vi "OneView.vi"() -> ()   [LabVIEW 2014]
uses:
  <vilib>/Utility/inputDevices.llb/keyboardAcquire.vi
  <vilib>/picture/3D Picture Control/NI_3D Picture Control.lvlib
  <vilib>/picture/3D Picture Control/Object/Create Object (name).vi
panel:
  out "View":refnum<vi>(3d-picture)
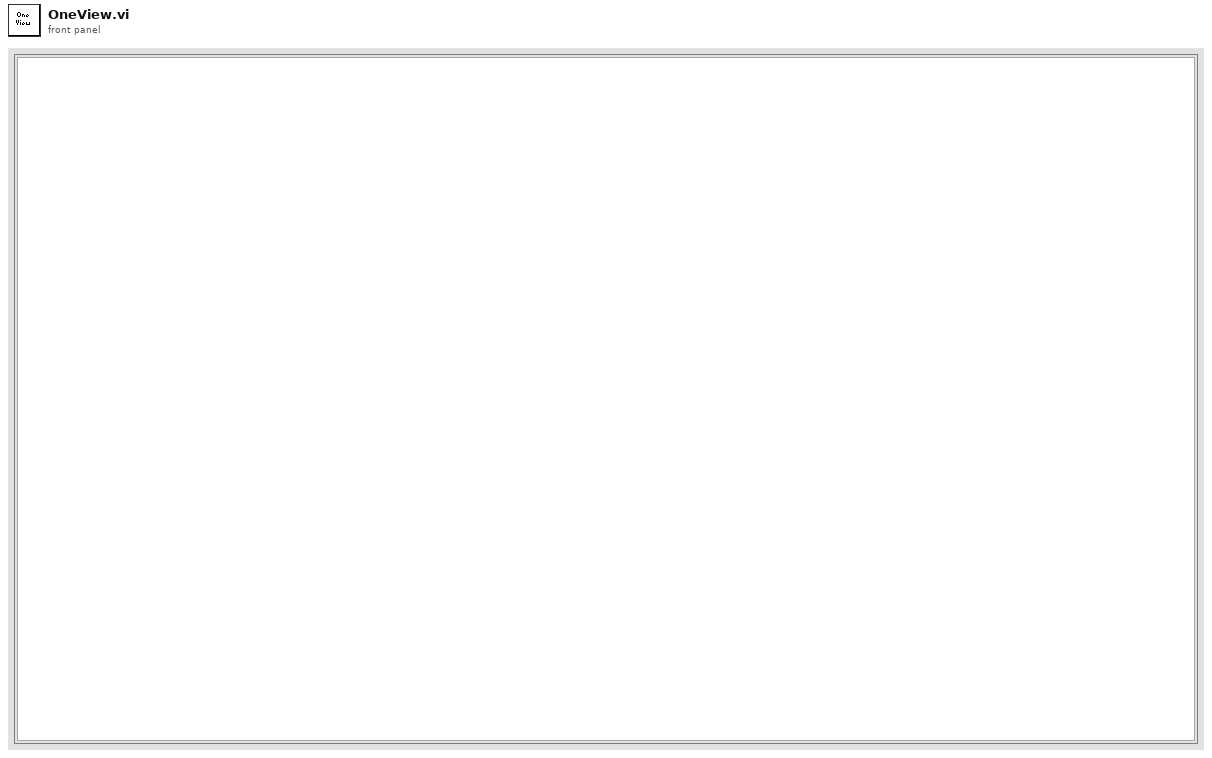
[diagram p1: front panel]
types:
  T1 = enum16{"None", "Spherical", "Flying", "Oriented"}
  T2 = enum16{"0", "1", "2", "3", "4", "5", "6", "7", "8", "9", "A", "B", "C", "D", "E", "F", "G", "H", "I", "J", "K", "L", "M", "N", "O", "P", "Q", "R", "S", "T", "U", "V", "W", "X", "Y", "Z", "F1", "F2", "F3", "F4", "F5", "F6", "F7", "F8", "F9", "F10", "F11", "F12", "F13", "F14", "F15", "ADD", "BACK", "BACKSLASH", "CAPITAL", "COMMA", "DECIMAL", "DELETE", "DIVIDE", "DOWN", "END", "EQUALS", "ESCAPE", "GRAVE (`)", "HOME", "INSERT", "LBRACKET", "LCONTROL", "LEFT", "L ALT", "LSHIFT", "LWIN", "MINUS", "MULTIPLY", "NEXT", "NUMLOCK", "NUMPAD_0", "NUMPAD_1", "NUMPAD_2", "NUMPAD_3", "NUMPAD_4", "NUMPAD_5", "NUMPAD_6", "NUMPAD_7", "NUMPAD_8", "NUMPAD_9", "PAUSE", "PERIOD", "PRIOR (PG UP)", "RBRACKET", "RCONTROL", "RETURN", "RIGHT", "R ALT", "RSHIFT", "RWIN", "SCROLL", "SEMICOLON", "SLASH", "SPACE", "SUBTRACT", "TAB", "UP", "ENTER (num pad)", "' (quote)"}
  T3 = typedef "lveventtype.ctl" = enum32{"Null", "Timeout", "Annotation Menu Selection", "Annotation Menu Selection?", "App Instance Close", "App Instance Close?", "Autoscale Range Change", "Bookmark Info Change", "Cell Edit", "Cell Edit?", "Cursor Grab", "Cursor Grab?", "Cursor Menu Selection", "Cursor Menu Selection?", "Cursor Move", "Cursor Release", "Data Change", "Direction Change", "Display State Change", "Drag Ended", "Drag Enter", "Drag Leave", "Drag Over", "Drag Source Update", "Drag Starting", "Drag Starting?", "Drop", "Exec State Change", "Key Down", "Key Down?", "Key Repeat", "Key Repeat?", "Key Up", "Listbox Double Click", "Menu Activation?", "Menu Selection (App)", "Menu Selection? (App)", "Menu Selection (User)", "Mouse Down", "Mouse Down?", "Mouse Enter", "Mouse Leave", "Mouse Move", "Mouse Up", "Mouse Wheel", "NI Security User Change (App)", "Pane Size", "Panel Close", "Panel Close?", "Panel Resize", "Plot Attribute Change", "Scale Range Change", "Shortcut Menu Activation?", "Shortcut Menu Selection (App)", "Shortcut Menu Selection? (App)", "Shortcut Menu Selection (User)", "Tree Double Click", "Tree Drag", "Tree Drag?", "Tree Drop", "Tree Drop?", "Tree Item Close", "Tree Item Close?", "Tree Item Open", "Tree Item Open?", "User Event", "Value Change"}
  T4 = typedef "LVPoint32TypeDef.ctl" = cluster{"Horizontal":i32, "Vertical":i32}
  T5 = enum16{"0", "1", "2", "3", "4", "5", "6", "7", "8", "9", "A", "B", "C", "D", "E", "F", "G", "H", "I", "J", "K", "L", "M", "N", "O", "P", "Q", "R", "S", "T", "U", "V", "W", "X", "Y", "Z", "F1", "F2", "F3", "F4", "F5", "F6", "F7", "F8", "F9", "F10", "F11", "F12", "F13", "F14", "F15", "ADD", "BACK", "BACKSLASH", "CAPITAL", "COMMA", "DECIMAL", "DELETE", "DIVIDE", "DOWN", "END", "EQUALS", "ESCAPE", "GRAVE (`)", "HOME", "INSERT", "LBRACKET", "LCONTROL", "LEFT", "L ALT", "LSHIFT", "LWIN", "MINUS", "MULTIPLY", "NEXT", "NUMLOCK", "NUMPAD_0", "NUMPAD_1", "NUMPAD_2", "NUMPAD_3", "NUMPAD_4", "NUMPAD_5", "NUMPAD_6", "NUMPAD_7", "NUMPAD_8", "NUMPAD_9", "PAUSE", "PERIOD", "PRIOR (PG UP)", "RBRACKET", "RCONTROL", "RETURN", "RIGHT", "R ALT", "RSHIFT", "RWIN", "SCROLL", "SEMICOLON", "SLASH", "SPACE", "SUBTRACT", "TAB", "UP", "ENTER (num pad)", "' (quote)"}[]
  T6 = typedef "Camera.ctl" = cluster{"Camera Position":T7, "Target":T7, "Up Direction":T7}
  T7 = typedef "LV3DPointTypeDef.ctl" = cluster{"X":sgl, "Y":sgl, "Z":sgl}
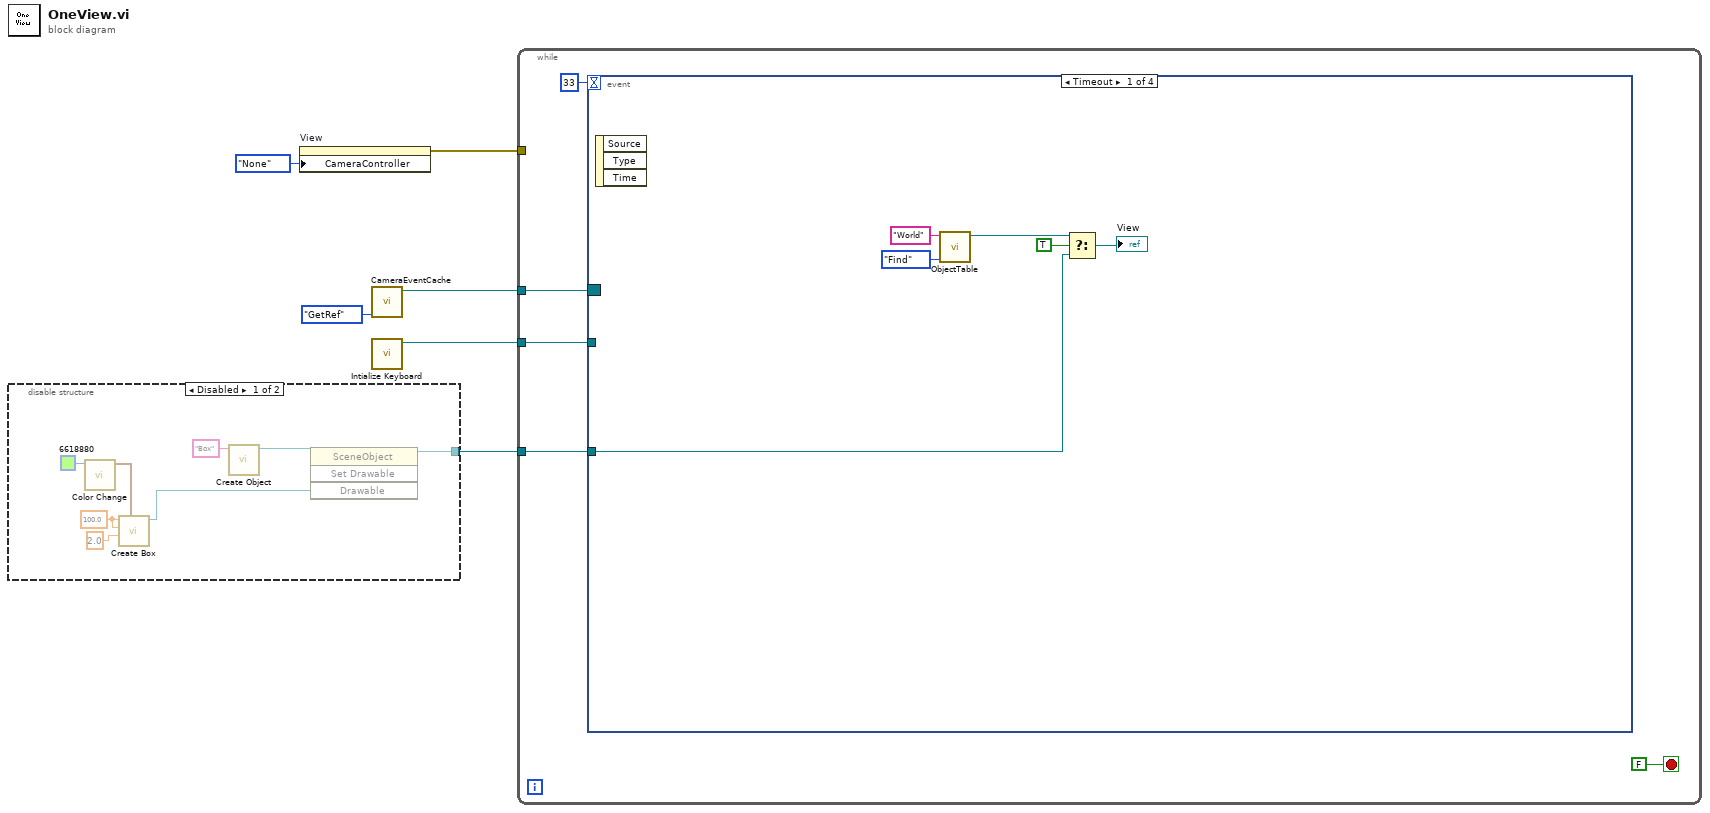
[diagram p0: block diagram]
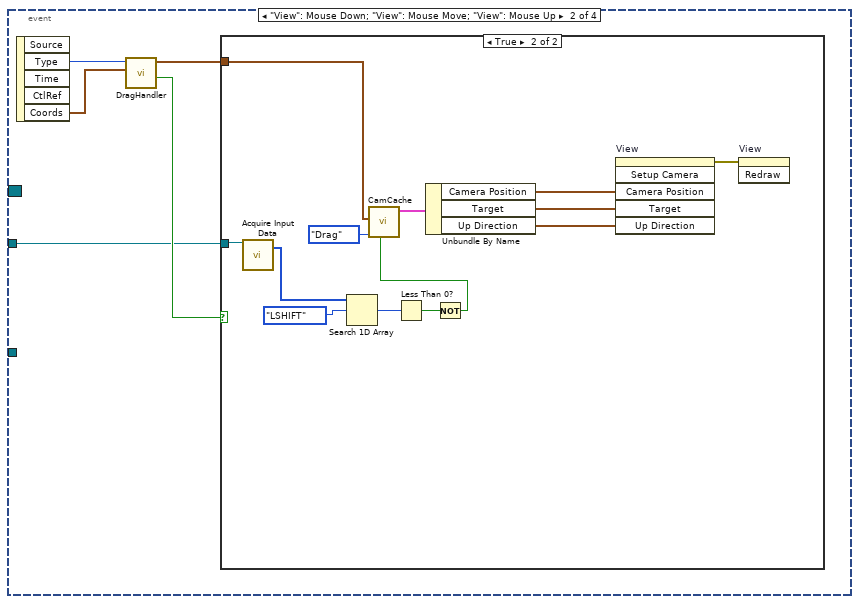
[diagram p3: hidden frame]
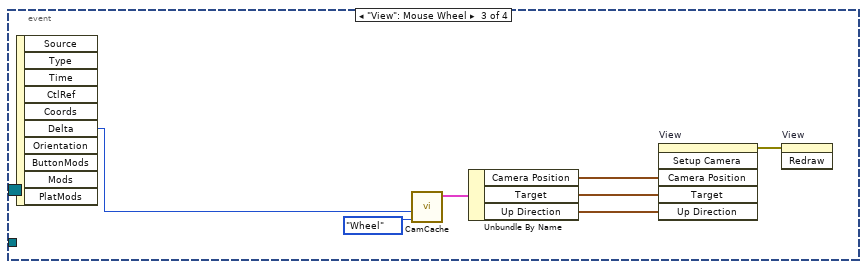
[diagram p5: hidden frame]
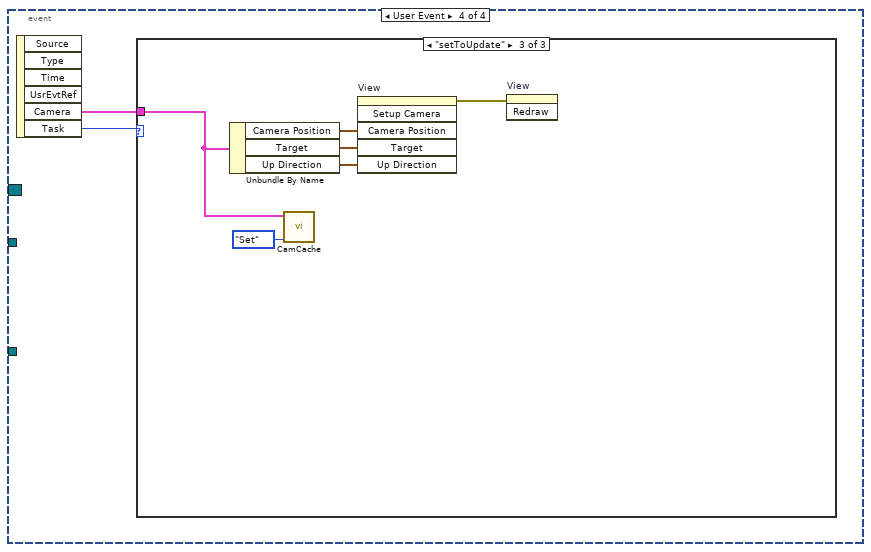
[diagram p6: hidden frame]
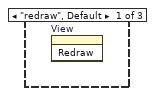
[diagram p7: hidden frame]
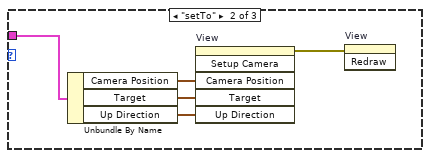
[diagram p8: hidden frame]
diagram:
  n1 = disable-structure shown="Disabled" {
    disable-tunnel: [w7 _] -> w4
    frame Disabled {
      w14 = sgl 100.0 ("Length X")
      n2 = call <vilib>:"Color Change.vi"("Color"=u32 6618880) -> ("RGBA"=w11:cluster{"R":sgl, "G":sgl, "B":sgl, "A":sgl})  [unwired: 10 in]
      n3 = call <vilib>:"Create Box.vi"("Color"=w11, "Length Z"=sgl 2.0, "Length Y"=w14, "Length X"=w14) -> ("New Box Refnum"=w8:refnum<vi>)  [unwired: 6 in, 1 out]
      n4 = call-poly <vilib>:"Create Object.vi"("Name"="Box") -> ("Scene:New Object"=w9:refnum<vi>)  [unwired: 9 in, 1 out]
      n5 = invoke class="SceneObject" method="Set Drawable"(reference=w9, "Drawable"=w8) -> (reference out=w7:refnum<vi>)  [unwired: 2 in, 3 out]
    }
    frame Enabled {
    }
  }
  n6 = property on="View" class="SceneGraphDisp (strict)"("CameraController"=T1."None" ("Camera Controller:Type")) -> (error out=w5:errorcluster)  [unwired: 2 in, 1 out]
  n7 = call "CameraEventCache.vi"("Operation"=enum16{"Create", "GetRef", "Fire"}."GetRef") -> ("EventRef"=w2:refnum<event-registration>)  [unwired: 10 in]
  n8 = call <vilib>:"Intialize Keyboard.vi"() -> ("device ID"=w1:refnum<k1>)  [unwired: 10 in, 1 out]
  n9 = while {
    tunnel: w5 -> [_]
    tunnel: w4 -> [w17]
    tunnel: w2 -> [w16]
    tunnel: w1 -> [w15]
    stop <- FALSE stop-if-true
    n10 = event shown="[0] Timeout" {
      selector: w16 -> [_ _ _ _]
      dyn-events: _ -> [_ _ _ _]
      timeout: 33 -> [_ _ _ _]
      tunnel: w17 -> [w23 _ _ _]
      tunnel: w15 -> [_ w26 _ _]
      event Timeout {
        n11 = event-data() -> ()  [unwired: 1 in, 3 out]
        n12 = call "ObjectTable.vi"("ObjectStoreSelector"=enum16{"New", "Find", "FindPattern", "GetTable"}."Find", "Name"="World") -> ("ObjectRef"=w22:refnum<vi>)  [unwired: 5 in, 4 out]
        n13 = Select(t=w22, s=TRUE, f=w23) -> (s? t:f=→"View":refnum<vi>)
      }
      event "View": Mouse Down; "View": Mouse Move; "View": Mouse Up {
        n14 = event-data() -> ("Type"=w30:T3, "Coords"=w29:T4)  [unwired: 1 in, 3 out]
        n15 = call "DragHandler.vi"("Coords"=w29, "Type"=w30) -> ("ValidDrag?"=w28:bool, "IncDrag"=w27:cluster{"X Cen":dbl, "Y Cen":dbl})  [unwired: 8 in]
        n16 = case shown="True" w28 {
          tunnel: w27 -> [_ w42]
          tunnel: w26 -> [_ w36]
          frame False {
          }
          frame True {
            n17 = call-poly <vilib>:"Acquire Input Data.vi"("device ID"=w36) -> ("keys pressed"=w35:T5)  [unwired: 16 in, 2 out]
            n18 = Search 1D Array(1D array=w35, element=T2."LSHIFT" ("keyType 3")) -> (index of element=w33:i32)  [unwired: 1 in]
            n19 = Less Than 0?(x=w33) -> (x < 0?=w32:bool)
            n20 = Not(x=w32) -> (.not. x?=w31:bool)
            n21 = call "CamCache.vi"("Shift"=w31, "Operation"=enum16{"Set", "Get", "Wheel", "Drag"}."Drag", "IncDrag"=w42) -> ("CamOut"=w40:T6)  [unwired: 8 in]
            n22 = Unbundle By Name(w40) -> ("Camera Position"=w39:T7, "Target"=w38:T7, "Up Direction"=w37:T7)
            n23 = invoke on="View" class="SceneGraphDisp (strict)" method="Setup Camera"("Camera Position"=w39, "Target"=w38, "Up Direction"=w37) -> (error out=w43:errorcluster)  [unwired: 3 in, 5 out]
            n24 = invoke on="View" class="SceneGraphDisp (strict)" method="Redraw"(error in=w43) -> ()  [unwired: 2 in, 3 out]
          }
        }
      }
      event "View": Mouse Wheel {
        n25 = event-data() -> ("Delta"=w44:i32)  [unwired: 1 in, 9 out]
        n26 = call "CamCache.vi"("Operation"=enum16{"Set", "Get", "Wheel", "Drag"}."Wheel", "Delta"=w44) -> ("CamOut"=w48:T6)  [unwired: 9 in]
        n27 = Unbundle By Name(w48) -> ("Camera Position"=w47:T7, "Target"=w46:T7, "Up Direction"=w45:T7)
        n28 = invoke on="View" class="SceneGraphDisp (strict)" method="Setup Camera"("Camera Position"=w47, "Target"=w46, "Up Direction"=w45) -> (error out=w50:errorcluster)  [unwired: 3 in, 5 out]
        n29 = invoke on="View" class="SceneGraphDisp (strict)" method="Redraw"(error in=w50) -> ()  [unwired: 2 in, 3 out]
      }
      event User Event {
        n30 = event-data() -> ("Camera"=w51:T6, "Task"=w52:enum16{"redraw", "setTo", "setToUpdate"})  [unwired: 1 in, 4 out]
        n31 = case shown="\"setToUpdate\"" w52 {
          tunnel: w51 -> [_ w57 w59]
          frame "redraw", Default {
            n32 = invoke on="View" class="SceneGraphDisp (strict)" method="Redraw"() -> ()  [unwired: 3 in, 3 out]
          }
          frame "setTo" {
            n33 = Unbundle By Name(w57) -> ("Camera Position"=w56:T7, "Target"=w55:T7, "Up Direction"=w54:T7)
            n34 = invoke on="View" class="SceneGraphDisp (strict)" method="Setup Camera"("Camera Position"=w56, "Target"=w55, "Up Direction"=w54) -> (error out=w53:errorcluster)  [unwired: 3 in, 5 out]
            n35 = invoke on="View" class="SceneGraphDisp (strict)" method="Redraw"(error in=w53) -> ()  [unwired: 2 in, 3 out]
          }
          frame "setToUpdate" {
            n36 = Unbundle By Name(w59) -> ("Camera Position"=w63:T7, "Target"=w62:T7, "Up Direction"=w61:T7)
            n37 = call "CamCache.vi"("Operation"=enum16{"Set", "Get", "Wheel", "Drag"}."Set", "CamIn"=w59) -> ()  [unwired: 9 in, 1 out]
            n38 = invoke on="View" class="SceneGraphDisp (strict)" method="Setup Camera"("Camera Position"=w63, "Target"=w62, "Up Direction"=w61) -> (error out=w60:errorcluster)  [unwired: 3 in, 5 out]
            n39 = invoke on="View" class="SceneGraphDisp (strict)" method="Redraw"(error in=w60) -> ()  [unwired: 2 in, 3 out]
          }
        }
      }
    }
  }
